vi "Main.vi"() -> ()   [LabVIEW 2013] (continued)
              tunnel: DB_-_[TransactionNo],[OrderNo]."h.[AdditionalProcs]" ("h.[TransactionNo],i.[OrderNo]\n2014-09-27 11:16") -> [w2623]
              tunnel: w2507 -> [w2613]
              tunnel: w2550 -> [w2622]
              tunnel: w2508 -> [w2606]
              tunnel: w2505 -> [w2604]
              tunnel: w2504 -> [w2602]
              tunnel: w2526 -> [w2621]
              tunnel: w2532 -> [w2620]
              tunnel: w2525 -> [w2619]
              tunnel: DB_-_[TransactionNo],[OrderNo]."h.[OutputSetId]" ("h.[TransactionNo],i.[OrderNo]\n2014-09-27 11:16") -> [w2616]
              tunnel: "Output Set" ("String") -> [w2611]
              tunnel: [w2610] -> w2518
              tunnel: w2501 -> [w2600]
              tunnel: [w2598] -> w2500 mode=indexing
              tunnel: w2499 -> [w2597]
              # "8"
              # "SpreadsheetString has \\r\\n\notherwise must add \\r\\n"
              # "6"
              # "4"
              # "7"
              # "Parameters"
              # "9"
              # "3"
              # "2"
              # "1"
              # "Each Order No"
              n1506 = for {
                tunnel: w2617 -> [w2657]
                tunnel: w2624 -> [w2656] mode=indexing
                shift-right: [w2651] -> w2615
                shift-left: w2597 -> [w2655]
                tunnel: w2621 -> [w2654] mode=indexing
                # "Part Details Columns"
                n1507 = Index Array(array=w2657, index=w2656) -> (element=w2653:string)
                n1508 = Build Array "Col0\nCol1"(w2654, w2653) -> (w2652:string[])
                n1509 = Build Array (concatenate) "New Row"(w2655, w2652) -> (w2651:string[][])
              }
              n1510 = Build Array (concatenate) "New Rows"(w2615, w2614, w2613) -> (w2612:string[][])
              n1511 = for {
                tunnel: w2617 -> [w2650]
                tunnel: w2622 -> [w2649] mode=indexing
                shift-right: [w2644] -> w2618
                shift-left: w2612 -> [w2646]
                tunnel: w2620 -> [w2648] mode=indexing
                # "WPS Column"
                n1512 = Index Array(array=w2650, index=w2649) -> (element=w2647:string)
                n1513 = Build Array "Col0\nCol1"(w2648, w2647) -> (w2645:string[])
                n1514 = Build Array (concatenate) "New Row"(w2646, w2645) -> (w2644:string[][])
              }
              n1515 = flat-sequence {
                tunnel: w2623 -> [w2636]
                tunnel: w2617 -> [w2635]
                tunnel: w2619 -> [w2634]
                tunnel: [w2631] -> w2609
                tunnel: w2618 -> [w2633]
                frame #0 {
                  # "5"
                  # "Additional WPS Column"
                  n1516 = Index Array(array=w2635, index=w2636) -> (element=w2630:string)
                  n1517 = Spreadsheet String To Array(delimiter (Tab)="\r\n", format string="", spreadsheet string=w2630, array type (2D Dbl)=string[] []) -> (array=w2626:string[])
                  n1518 = for {
                    tunnel: w2626 -> [w2639] mode=indexing
                    tunnel: [w2639] -> w2625 mode=indexing if=w2637
                    n1519 = Search and Replace String(replace all?=TRUE ("replace all? (F)"), input string=w2639, search string=",") -> (result string=w2641:string)  [unwired: 5 in, 3 out]
                    n1520 = call <vilib>:"Trim Whitespace.vi"("string"=w2641) -> ("trimmed string"=w2640:string)  [unwired: 1 in]
                    n1521 = Empty String/Path?(string/path=w2640) -> (empty?=w2638:bool)
                    n1522 = Not(x=w2638) -> (.not. x?=w2637:bool)
                  }
                  n1523 = Build Array (concatenate) "Col0\nCol1"(w2634, w2625) -> (w2632:string[])
                  n1524 = Build Array (concatenate) "New Row"(w2633, w2632) -> (w2631:string[][])
                }
              }
              n1525 = Index Array(array=w2617, index=w2616) -> (element=w2610:string)
              n1526 = Build Array "Col0\nCol1"(w2611, w2610) -> (w2608:string[])
              n1527 = Build Array (concatenate) "New Row"(w2609, w2608) -> (w2607:string[][])
              n1528 = Build Array (concatenate) "New Rows"(w2607, w2606) -> (w2605:string[][])
              n1529 = Build Array (concatenate) "New Row"(w2605, w2604) -> (w2603:string[][])
              n1530 = Build Array (concatenate) "New Row"(w2603, w2602) -> (w2601:string[][])
              n1531 = Build Array (concatenate) "New Row"(w2601, w2600) -> (w2599:string[][])
              n1532 = Flatten To String(anything=w2599) -> (data string=w2598:string)  [unwired: 3 in, 2 out]
            }
            n1533 = call "DB - [MasterData].[OutputSet].vi"("Master Data OuputSet SQL"=DB_-_Master_Data_OutputSet_SQL."SELECT [LayoutFilePath],[LayoutFileName]", "[PlantId]"=w2521, "[OutputSetId]"=w2518) -> ("Template Files"=w2517:string[], "[LayoutId]"=w2515:string[])  [unwired: 4 in, 3 out]
            n1534 = String To Path(string=w2517) -> (path=w2516:path[])
            n1535 = local write "DB"(w2533) -> ()
          }
        }
        "Order No" <- w2205
        "Details From .stp and Parameters" <- w2210
        n1536 = Array Size(array=w2205) -> (size(s)=w2206:i32)
        "No Of Orders" <- w2206
        n1537 = local read "DB - Report"() -> (w2199:bool)
        n1538 = Format Date/Time String "Date_Time"(time format string (%c)="%Y%m%d_%H%M%S") -> (date/time string=w2203:string)  [unwired: 2 in]
        n1539 = Format Into String(format string="%02d", w2206) -> (resulting string=w2201:string)  [unwired: 2 in, 1 out]
        n1540 = local read "Chart Separation by Order#"() -> (w2204:bool)
        n1541 = case shown="True" w2199 {
          tunnel: w2197 -> [_ w2379]
          tunnel: w2173 -> [_ w2377]
          tunnel: ["00" ("[ReportRunNo]") w2372] -> w2198
          tunnel: [w2356 w2361] -> w2172
          tunnel: [w2355 w2360] -> w2171
          frame False {
            # "Use Logon's INFO if no Database"
            n1542 = local read "Logon (Report Buffer)"() -> (w2357:T21)
            n1543 = Unbundle By Name(w2357) -> ("PlantID"=w2356:string, "SystemID"=w2355:string)
          }
          frame True {
            w2362 = 1  # [SystemId]
            w2363 = 0  # [PlantId]
            w2378 = ""  # Not Needed for [TransactionRunNo]
            # "[Execute].[TransactionReport] logged inside subVI"
            n1544 = Bundle("TransactionNo"=w2379, "Not Needed for [TransactionRunNo]"=w2378) -> (w2365:T67)  [unwired: 1 in]
            n1545 = call "DB - [Execute].[ReportList].vi"(2:DB_-_Execute_ReportList_Enum."INSERT INTO [Execute].[TransactionReport]", "Transaction"=w2365, "error in (no error)"=w2377) -> ("[ReportRunNo]"=w2373:string, "SUMMARY"=w2369:errorcluster)  [unwired: 9 in, 2 out]
            n1546 = Concatenate Strings("{Report Generate Toggle} [ReportRunNo] = " ("Message"), w2373) -> (w2370:string)
            n1547 = local read "Transaction (Report Buffer)"() -> (w2359:T19)
            n1548 = Decimal String To Number(string=w2373) -> (number=w2374:i32)  [unwired: 2 in, 1 out]
            n1549 = call "Queue - EnQueue to MessageQ.vi"("<NoD> Don't Display to UI"=TRUE, "Message"=w2370) -> ()  [unwired: 9 in, 1 out]
            n1550 = Format Into String(format string="%02d", w2374) -> (resulting string=w2372:string)  [unwired: 2 in, 1 out]
            n1551 = call "DB - [Setup].[Item] (Part Details).vi"("DB - Setup Item Enum"=DB_-_Setup_Item_Enum."SELECT [EquipmentxId]", "DB.Schema.Table Array"=string[] ["SRTRS.Execute.Header"], "Transaction"=w2359, "error in (no error)"=w2369) -> ("1D Results"=w2364:string[], "SUMMARY"=w2368:errorcluster)  [unwired: 6 in, 4 out]
            n1552 = Index Array(array=w2364, index #1=w2363, index #2=w2362) -> (element #1=w2361:string, element #2=w2360:string)
            n1553 = local write "DB"(w2368) -> ()
          }
        }
        n1554 = Concatenate Strings(w2201, w2198) -> (w2208:string)
        n1555 = Select(t=w2208, s=w2204, f=w2203) -> (s? t:f=w2202:string)
        n1556 = flat-sequence {
          tunnel: w2200 -> [w2352]
          tunnel: [w2352] -> w2196
          frame #0 {
            n1557 = call "Msgbox - Add OR Remove.vi"("MsgBox"=T44 {"Show"=FALSE, "Priority"=0, "Message"="Report Generation...(Done)", "seconds"=30}) -> ("Error Out"=→"Msgbox":errorcluster)  [unwired: 9 in, 1 out]
          }
        }
        n1558 = for {
          tunnel: [w2245] -> w2179 mode=concatenating
          tunnel: w2210 -> [w2244]
          tunnel: w2205 -> [w2243]
          tunnel: w2202 -> [w2242]
          tunnel: w2201 -> [w2241]
          tunnel: [w2240] -> w2193
          tunnel: w2198 -> [w2238]
          tunnel: w2197 -> [w2237]
          shift-right: [w2239] -> w2200
          shift-left: w2173 -> [w2235]
          tunnel: w2195 -> [w2234] mode=indexing
          tunnel: w2194 -> [w2233] mode=indexing
          tunnel: w2172 -> [w2232]
          tunnel: w2171 -> [w2231]
          i -> [w2236]
          # "Template Files"
          n1559 = local write "Template File"(w2234) -> ()
          n1560 = local write "Layout ID"(w2233) -> ()
          n1561 = for {
            tunnel: w2244 -> [w2284] mode=indexing
            tunnel: w2243 -> [w2268] mode=indexing
            tunnel: w2237 -> [w2269]
            tunnel: w2242 -> [w2286]
            shift-right: [w2283] -> w2239
            shift-left: w2235 -> [w2253]
            tunnel: [w2280] -> w2245 mode=indexing
            tunnel: w2238 -> [w2248]
            tunnel: w2241 -> [w2267]
            tunnel: [w2264] -> w2240
            tunnel: w2234 -> [w2262]
            tunnel: w2236 -> [w2258]
            tunnel: w2233 -> [w2260]
            tunnel: w2232 -> [w2247]
            tunnel: w2231 -> [w2246]
            i -> [w2259]
            w2282 = "\"" ("string")
            w2261 = "_" ("string")
            # "List by Order Number (Easier to maintain code if on seperate loop)"
            n1562 = Equal To 0?(x=w2258) -> (x = 0?=w2256:bool)
            n1563 = Equal To 0?(x=w2259) -> (x = 0?=w2257:bool)
            n1564 = And(x=w2257, y=w2256) -> (x .and. y?=w2255:bool)
            n1565 = local read "Excel"() -> (w2263:path)
            n1566 = local read "Reports"() -> (w2274:path)
            n1567 = Concatenate Strings(w2260, w2261, w2269, w2261, w2268, w2261, w2286, ".xls" ("string")) -> (w2254:string)
            n1568 = case shown="True" w2255 {
              frame True {
                n1569 = call "Msgbox - Add OR Remove.vi"("MsgBox"=T44 {"Show"=TRUE, "Priority"=0, "Message"="Report Generation...", "seconds"=30}) -> ("Error Out"=w2288:errorcluster)  [unwired: 9 in, 1 out]
                n1570 = local write "Msgbox"(w2288) -> ()
              }
              frame False {
              }
            }
            n1571 = call "Folder - Create Year-Month.vi"("error in (no error)"=w2253, "Folder Name"=w2274) -> ("error out"=w2276:errorcluster, "Folder with Year\\Month"=w2266:path)  [unwired: 8 in]
            n1572 = call "Folder - Create Year-Month.vi"("error in (no error)"=w2253, "Folder Name"=w2263) -> ("error out"=w2277:errorcluster, "Folder with Year\\Month"=w2278:path)  [unwired: 8 in]
            n1573 = Merge Errors(w2277, w2276) -> (w2279:errorcluster)
            n1574 = local read "MasterData\\JPG"() -> (w2273:path)
            n1575 = local read "Raw Data File (Report Tab)"() -> (w2265:path)
            n1576 = Build Path(base path=w2278, name or relative path=w2254) -> (appended path=w2272:path)
            n1577 = local read "Logon"() -> (w2252:T21)
            n1578 = Unbundle By Name(w2252) -> ("LanguageID"=w2250:string)
            n1579 = local read "Temp_Host"() -> (w2271:path)
            n1580 = Bundle By Name(cluster=T50 {"[LanguageId]"="", "[ReportRunNo]"="", "[PlantId]"="", "[SystemId]"=""} ("Report Additional Details"), "[LanguageId]"=w2250, "[ReportRunNo]"=w2248, "[PlantId]"=w2247, "[SystemId]"=w2246) -> (w2249:T50)
            n1581 = Bundle("Reports"=w2274, "MasterData\\JPG"=w2273, "String"=w2262, "appended path"=w2272, "Raw Data File (Report Tab)"=w2265, "Temp_Host"=w2271) -> (w2270:T68)  [unwired: 1 in]
            "Report Files Cluster" <- w2270
            n1582 = while {
              tunnel: w2284 -> [w2302]
              tunnel: [w2297] -> w2283
              tunnel: w2279 -> [w2301]
              tunnel: w2270 -> [w2296]
              tunnel: w2249 -> [w2291]
              i -> [w2298]
              stop <- w2299 stop-if-true
              # "Try twice or no error"
              n1583 = local read "Chart Separation by Order#"() -> (w2294:bool)
              n1584 = local read "DB - Report"() -> (w2295:bool)
              n1585 = call "Report - Excel.vi"("pdf"="Report.Create.PDF", "Chart Seperation by Order#"=w2294, "Details from .stp and Parameters"=w2302, "Use DB for Picture (Material)"=w2295, "error in (no error)"=w2301, "Include MetaData"="Include MetaData", "Report Additional Details"=w2291, "Report Files Cluster"=w2296) -> ("error out"=w2300:errorcluster, "Picture Error"=w2290:errorcluster, "Material File"=w2289:string)  [unwired: 1 in]
              n1586 = case shown="Error" w2290 {
                tunnel: w2289 -> [_ w2303]
                frame No Error {
                }
                frame Error {
                  n1587 = Concatenate Strings("{Report} Pic Error:  " ("Message"), w2303) -> (w2304:string)
                  n1588 = call "Queue - EnQueue to MessageQ.vi"("<NoD> Don't Display to UI"=TRUE, "Message"=w2304) -> ()  [unwired: 9 in, 1 out]
                }
              }
              n1589 = case shown="Error" w2300 {
                selector: w2300 -> [w2307 w2309]
                tunnel: [TRUE w2310] -> w2299
                tunnel: w2298 -> [_ w2312]
                tunnel: [w2307 w2311] -> w2297
                frame No Error {
                }
                frame Error {
                  n1590 = Greater Or Equal?(x=w2312, y=2) -> (x >= y?=w2310:bool)
                  n1591 = case shown="True" w2310 {
                    tunnel: [errorcluster {"status"=FALSE, "code"=0, "source"=""} ("error out") w2315] -> w2311
                    tunnel: w2309 -> [_ w2315]
                    frame False {
                    }
                    frame True {
                    }
                  }
                }
              }
            }
            n1592 = Concatenate Strings(w2282, w2254, w2282) -> (w2281:string)
            n1593 = case shown="No Error" w2283 {
              tunnel: [_ " create ERROR." ("string")] -> w2275
              tunnel: w2268 -> [w2337 _]
              tunnel: w2248 -> [w2336 _]
              tunnel: w2267 -> [w2335 _]
              tunnel: w2266 -> [w2334 _]
              tunnel: w2265 -> [w2333 _]
              tunnel: [w2332 errorcluster {"status"=FALSE, "code"=0, "source"=""} ("SUMMARY")] -> w2264
              tunnel: w2254 -> [w2318 _]
              tunnel: w2260 -> [w2316 _]
              frame No Error {
                # "Use Logon or From Execute.Setup.Header?"
                n1594 = Search and Replace String(replace all?=TRUE ("replace all? (F)"), case sensitive?=TRUE ("ignore case? (F)"), input string=w2318, search string="xls", replace string="pdf" ("replace string (\"\")")) -> (result string=w2317:string)  [unwired: 3 in, 3 out]
                n1595 = Strip Path(path=w2333) -> (stripped path=w2324:path, name=w2323:string)
                n1596 = Path To String(path=w2334) -> (string=w2329:string)
                n1597 = Path To String(path=w2324) -> (string=w2325:string)
                n1598 = local read "ReportList Cluster"() -> (w2327:T18)
                n1599 = Bundle By Name(cluster=w2327, "[LayoutId]"=w2316, "[OrderNo]"=w2337, "[ReportRunNo]"=w2336, "[NoOfOrders]"=w2335, "[ReportFilePath]"=w2329, "[ReportFileName]"=w2317, "[RawDataSourcePath]"=w2325, "[RawDataSourceFileName]"=w2323) -> (w2328:T18)
                "ReportList Cluster" <- w2328
                n1600 = local read "Transaction (Report Buffer)"() -> (w2330:T19)
                n1601 = local read "Logon (Report Buffer)"() -> (w2326:T21)
                n1602 = call "DB - [Execute].[ReportList].vi"(2:DB_-_Execute_ReportList_Enum."INSERT INTO [Execute].[ReportList] ", "Transaction"=w2330, "ReportList Cluster"=w2328, "Logon"=w2326) -> ("SUMMARY"=w2332:errorcluster)  [unwired: 8 in, 3 out]
                n1603 = local write "DB"(w2332) -> ()
              }
              frame Error {
              }
            }
            n1604 = Concatenate Strings(w2281, w2275) -> (w2280:string)
          }
        }
        n1605 = case shown="True" w2199 {
          tunnel: w2200 -> [_ w2340]
          tunnel: w2198 -> [_ w2342]
          tunnel: w2197 -> [_ w2341]
          frame False {
            # "Skip DB"
          }
          frame True {
            # "Use DB - Update [ReportGenerateFail] Flag if Report Fail"
            n1606 = case shown="Error" w2340 {
              tunnel: w2342 -> [_ w2348]
              tunnel: w2341 -> [_ w2347]
              frame No Error {
              }
              frame Error {
                n1607 = Bundle("TransactionNo"=w2347, "") -> (w2345:cluster{"TransactionNo":string, string})  [unwired: 1 in]
                n1608 = call "DB - [Execute].[ReportList].vi"(2:DB_-_Execute_ReportList_Enum."UPDATE [Execute].[TransactionReport]", "[ReportGenerateFail]"=TRUE, "[ReportRunNo]"=w2348, "Transaction"=w2345) -> ("SUMMARY"=w2349:errorcluster)  [unwired: 8 in, 3 out]
                n1609 = local write "DB"(w2349) -> ()
              }
            }
          }
        }
        n1610 = Array To Spreadsheet String(delimiter (Tab)=", ", array=w2179, 3:"" ("format string")) -> (spreadsheet string=w2183:string)
        n1611 = Search and Replace String(replace all?=TRUE ("replace all? (F)"), case sensitive?=TRUE ("ignore case? (F)"), input string=w2183, search string="xls", replace string="pdf" ("replace string (\"\")")) -> (result string=w2182:string)  [unwired: 3 in, 3 out]
        n1612 = Search and Replace String(replace all?=TRUE ("replace all? (F)"), input string=w2182, search string="\r\n") -> (result string=w2178:string)  [unwired: 5 in, 3 out]
        n1613 = case shown="Error" w2196 {
          selector: w2196 -> [_ w2666]
          tunnel: ["<I 405>" ("<.?....> Message Code") "<E 406>" ("<.?....> Message Code")] -> w2192
          tunnel: ["Report Generate Successful" ("<.?....> Message Code") "Report Generate Fail" ("<.?....> Message Code")] -> w2191
          tunnel: [" report(s) Generated" ("<.?....> Message Code") "Please check output set and file server availability and Retry." ("<.?....> Message Code")] -> w2190
          tunnel: w2178 -> [w2658 _]
          tunnel: [w2658 _] -> w2177
          frame No Error {
            # "Report Generated OK!"
          }
          frame Error {
            # "Report Generate Failed."
            n1614 = Unbundle By Name(w2666) -> ("code"=w2665:i32)
            n1615 = case shown="0, Default" w2665 {
              tunnel: w2666 -> [_ _]
              frame 0, Default {
              }
              frame -8001 {
                # "Repeat?"
                # "Error Popup already shown\nearlier"
              }
            }
          }
        }
        n1616 = call "Msgbox - Message Handler.vi"("Short Description (When DB Not Available)"=w2191, "Description (When DB Not Available)"=w2190, "Pre-Description"=w2177, "<.?....> Message Code"=w2192) -> ("MHandler Error"=w2174:errorcluster)  [unwired: 5 in, 2 out]
        n1617 = local write "MHandler"(w2174) -> ()
        n1618 = case shown="No Error" w2193 {
          tunnel: ["<NoD>INSERT INTO [Execute].[ReportList]" ("Message") "Report List DB Error. /*INSERT [EXECUTE].[ReportList]*/" ("Message")] -> w2176
          frame No Error {
            # "No Need to Display this in Message."
          }
          frame Error {
          }
        }
        n1619 = call "Queue - EnQueue to MessageQ.vi"("<NoD> Don't Display to UI"=TRUE, "Message"=w2176) -> ()  [unwired: 9 in, 1 out]
        n1620 = flat-sequence {
          tunnel: w2193 -> [_]
          frame #0 {
            n1621 = local read "Template File"() -> (w2219:path)
            n1622 = local read "Layout ID"() -> (w2217:string)
            n1623 = Path To String(path=w2219) -> (string=w2216:string)
            n1624 = call <vilib>:"Application Directory.vi"() -> ("Application Directory"=w2224:path)
            n1625 = Concatenate Strings(w2217, "\t", w2216) -> (w2215:string)
            n1626 = Build Path(base path=w2224, name or relative path="SRTRS.ini" ("ini Name")) -> (appended path=w2223:path)
            n1627 = call <vilib>:"Open Config Data.vi"("create file if necessary (T)"=FALSE, "configuration file path"=w2223) -> ("error out"=w2226:errorcluster, "refnum"=w2225:T59)  [unwired: 7 in, 1 out]
            n1628 = call-poly <vilib>:"Write Key.vi"("write raw string? (F)"=TRUE, "section"="Settings", "error in (no error)"=w2226, "value"=w2215, "key"="Layout Details", "refnum"=w2225) -> ("error out"=w2230:errorcluster, "refnum out"=w2229:T59)  [unwired: 3 in, 1 out]
            n1629 = call <vilib>:"Close Config Data.vi"("error in (no error)"=w2230, "refnum"=w2229) -> ("error out"=w2228:errorcluster)  [unwired: 8 in, 1 out]
            n1630 = local write "ini File Error"(w2228) -> ()
          }
        }
      }
      event "------------------------------------        Simulate TAB      ------------------------------------": Value Change {
        n1631 = event-data() -> ()  [unwired: 1 in, 6 out]
      }
      event "Use Host COM Port": Value Change {
        # "Set COM Port to either Local PC or via cRIO"
        n1632 = event-data() -> ("CtlRef"=w2678:refnum<vi>)  [unwired: 1 in, 5 out]
        n1633 = property class="Bool (strict)"(reference=w2678) -> ("Label.Text"=w2676:string)  [unwired: 1 in, 2 out]
        n1634 = local read "Host COM Port"() -> (w2681:string)
        n1635 = local read "cRIO COM Port"() -> (w2680:string)
        n1636 = Select(t="TRUE.", s="Use Host COM Port", f="FALSE.") -> (s? t:f=w2671:string)
        n1637 = Concatenate Strings("{[" ("string"), w2676, "]}" ("string")) -> (w2674:string)
        n1638 = Select(t=w2681, s="Use Host COM Port", f=w2680) -> (s? t:f=w2679:string)
        n1639 = Concatenate Strings(w2674, " is Changed to " ("string"), w2671) -> (w2668:string)
        n1640 = local write "VISA resource name RS232"(w2679) -> ()
        n1641 = call "Queue - EnQueue to MessageQ.vi"("<NoD> Don't Display to UI"=TRUE, "Message"=w2668) -> ()  [unwired: 9 in, 1 out]
      }
      event "Simulate cRIO Started": Value Change {
        # "Seq Num        Ramp Rate       Target Temp        SegType"
        n1642 = event-data() -> ()  [unwired: 1 in, 6 out]
        n1643 = case shown="False" FALSE {
          tunnel: [100 ("Start Temp") 25 ("Start Temp")] -> w2685
          tunnel: [i32[][] [[2, 0, 0, 3], [3, 50, 80, 1], [4, 0, 0, 0]] ("Final Segments") i32[][] [[1, 100, 100, 1], [2, 0, 0, 3], [3, 50, 80, 1], [4, 0, 0, 0]] ("Final Segments")] -> w2684
          frame False {
            # "From Hold at 100° to Ramp Down"
          }
          frame True {
            # "All Segments (Ramp Up, Hold, Ramp Down)"
          }
        }
        n1644 = local read "cRIO shared variable RT Library"() -> (w2682:string)
        n1645 = control-ref of="cRIO Status"() -> (w2688:refnum<vi>)
        n1646 = call "cRIO - Shared Variable RW.vi"("shared variable RT Library"=w2682, "Read/Write"=cRIO_RW_Enum."Write", "Simulate cRIO"=TRUE, "Probe List In"=i32[] [1, 2], "DAQ Start"=TRUE, "cRIO Status"=w2688) -> ()  [unwired: 5 in, 9 out]
        n1647 = call "ET3500 - Simulate Profile.vi"("Popup"=FALSE, "Set (T) / Get (F)"=TRUE, "Start Temp"=w2685, "Final Segments"=w2684) -> ()  [unwired: 3 in, 5 out]
      }
      event "Data", "Excel", "Report.Create.Excel", "Report.Create.PDF", "Simulate cRIO", "Simulate ET3500": Value Change {
        # "<OPTIONS> are logged into MessageQ"
        n1648 = event-data() -> ("CtlRef"=w2706:refnum<vi>)  [unwired: 1 in, 5 out]
        n1649 = property class="Ctl"(reference=w2706) -> ("ClassName"=w2699:string, "Caption.Text"=w2700:string, "Value"=w2704:variant)  [unwired: 1 in, 2 out]
        n1650 = case shown="\"Boolean\"" w2699 {
          tunnel: w2704 -> [w2712 w2718]
          tunnel: [w2707 w2713] -> w2703
          frame "Path", Default {
            w2708 = "\"" ("string")
            n1651 = Variant To Data(type=path "", Variant=w2712) -> (data=w2710:path)  [unwired: 1 in, 1 out]
            n1652 = Path To String(path=w2710) -> (string=w2709:string)
            n1653 = Concatenate Strings(w2708, w2709, w2708) -> (w2707:string)
          }
          frame "Boolean" {
            n1654 = Variant To Data(type=TRUE, Variant=w2718) -> (data=w2716:bool)  [unwired: 1 in, 1 out]
            n1655 = Select(t="TRUE" ("string"), s=w2716, f="FALSE" ("string")) -> (s? t:f=w2713:string)
          }
        }
        n1656 = Concatenate Strings("<", w2700, ">", " changed to " ("string"), w2703) -> (w2698:string)
        n1657 = call "Queue - EnQueue to MessageQ.vi"("<NoD> Don't Display to UI"=TRUE, "Message"=w2698) -> ()  [unwired: 9 in, 1 out]
      }
      event "------------------------------------        MCListBox       ------------------------------------": Value Change {
        n1658 = event-data() -> ()  [unwired: 1 in, 6 out]
      }
      event "MCListBox FHS Setup Add Button", "MCListBox FHS Setup Remove Button", "MCListBox AWPS Add Button", "MCListBox AWPS Remove Button", "MCListBox FHS Master Data Add Button", "MCListBox FHS Master Data Remove Button": Value Change {
        # "New and Unsed Cells have same color for\nAWPS but different color for FHS Master Data"
        # "Not in used"
        n1659 = event-data() -> ("CtlRef"=w2733:refnum<vi>)  [unwired: 1 in, 5 out]
        n1660 = local read "CellBG Unused Cells"() -> (w2725:u32)
        n1661 = local read "CellBG New Cells"() -> (w2726:u32)
        n1662 = Or(x="MCListBox FHS Master Data Add Button", y="MCListBox FHS Master Data Remove Button") -> (x .or. y?=w2720:bool)
        n1663 = Or(x="MCListBox FHS Setup Add Button", y="MCListBox FHS Setup Remove Button") -> (x .or. y?=w2721:bool)
        n1664 = Or(x=w2721, y=w2720) -> (x .or. y?=w2719:bool)
        n1665 = Select(t=w2726, s=w2719, f=w2725) -> (s? t:f=w2724:u32)
        n1666 = case shown="True" "MCListBox AWPS Add Button" {
          tunnel: [T5[] [] w2753] -> w2732
          tunnel: [_ w2752] -> w2730
          frame False {
          }
          frame True {
            w2747 = ""
            # "To Add via ComboBox"
            n1667 = control-ref of="Additional Rev"() -> (w2754:refnum<vi>)
            n1668 = control-ref of="Additional WPS/Ref"() -> (w2755:refnum<vi>)
            n1669 = control-ref of="MCListBox AWPS"() -> (w2746:refnum<vi>)
            n1670 = property class="MCListbox (strict)"(reference=w2746) -> ("ItemNames"=w2745:string[][])  [unwired: 1 in, 2 out]
            n1671 = property class="CmbBox (strict)"(reference=w2755) -> (reference out=w2749:refnum<vi>, "Value"=w2743:T5)  [unwired: 1 in, 1 out]
            n1672 = property class="CmbBox (strict)"(reference=w2754) -> (reference out=w2748:refnum<vi>, "Value"=w2736:T5)  [unwired: 1 in, 1 out]
            n1673 = Array To Spreadsheet String(array=w2745, 3:"" ("format string")) -> (spreadsheet string=w2739:string)  [unwired: 1 in]
            n1674 = Empty String/Path?(string/path=w2736) -> (empty?=w2750:bool)
            n1675 = call <vilib>:"Space Constant.vi"() -> ("String"=w2735:string)
            n1676 = Select(t=w2735, s=w2750, f=w2736) -> (s? t:f=w2741:T5)
            n1677 = Empty String/Path?(string/path=w2743) -> (empty?=w2751:bool)
            n1678 = Concatenate Strings(w2743, "\\t", w2741) -> (w2740:string)
            n1679 = Match Pattern(string=w2739, regular expression=w2740) -> (offset past match=w2738:i32)  [unwired: 1 in, 3 out]
            n1680 = Greater Or Equal To 0?(x=w2738) -> (x >= 0?=w2737:bool)
            n1681 = Build Array(w2743, w2741) -> (w2753:T5[])
            n1682 = case shown="True" w2751 {
              tunnel: [w2756 errorcluster {"status"=TRUE, "code"=0, "source"=""} ("error constant")] -> w2752
              tunnel: w2737 -> [w2757 _]
              frame False {
                # "Not Empty Field"
                n1683 = case shown="True" w2757 {
                  tunnel: [_ errorcluster {"status"=TRUE, "code"=0, "source"=""} ("error constant")] -> w2756
                  frame False {
                  }
                  frame True {
                    # "Addtional WPS and Rev already Exists in AWPS MCListBox"
                    n1684 = call "Msgbox - Format Message.vi"("Message"="Duplicates. Additional WPS/Ref and Rev are not Added." ("message"), "Message Code\n2014-10-01"=Message_Code_-_Enum."<APP><W 130>" ("Message Code\n2014-10-01")) -> ("Message"=w2760:string)  [unwired: 8 in, 1 out]
                    n1685 = call "Msgbox UI.vi"("[MessageType]"=w2760) -> ()  [unwired: 8 in, 3 out]
                  }
                }
              }
              frame True {
                # "Empty Field"
                n1686 = call "Msgbox - Format Message.vi"("Message"="Empty Field. Additional WPS/Ref and Rev are not Added." ("message"), "Message Code\n2014-10-01"=Message_Code_-_Enum."<APP><W 130>" ("Message Code\n2014-10-01")) -> ("Message"=w2764:string)  [unwired: 8 in, 1 out]
                n1687 = call "Msgbox UI.vi"("[MessageType]"=w2764) -> ()  [unwired: 8 in, 3 out]
              }
            }
            n1688 = property class="CmbBox (strict)"(reference=w2749, "Value"=w2747) -> ()  [unwired: 1 in, 2 out]
            n1689 = property class="CmbBox (strict)"(reference=w2748, "Value"=w2747) -> ()  [unwired: 1 in, 2 out]
          }
        }
        n1690 = call "MCListbox Event - Add and Remove Buttons.vi"("CellBG New Cells"=w2724, "CellBG Unused Cells"=w2725, "new element/subarray"=w2732, "Error In"=w2730, "MCListBox Ref"=w2731, "CtlRef Boolean"=w2733) -> ()  [unwired: 5 in, 1 out]
      }
      event "MCListBox FHS Setup", "MCListBox FHS Master Data": Key Down? {
        # "Only the 2 FHS (Furnace Heating Sequence) have direct Keyboard Entries"
        n1691 = event-data() -> ("CtlRef"=w2767:refnum<vi>, "Char"=w2768:i16, "VKey"=w2770:T55)  [unwired: 1 in, 7 out]
        n1692 = property class="MCListbox (strict)"(reference=w2767) -> ("EditPos"=w2766:T33)  [unwired: 1 in, 2 out]
        n1693 = call "MCListbox Event - Key Down QuestionMark.vi"("Key Down?"=w2772, "CtlRef"=w2767) -> ()  [unwired: 9 in, 1 out]
        n1694 = case "Only NUMBERS, BackSpace and (Return, Enter, Up, Down, Right, Left, Delete)" shown="8, 46, 48..57" w2768 {
          tunnel: [w2774 w2777 w2778] -> w2769
          tunnel: w2770 -> [w2773 _ _]
          tunnel: w2766 -> [_ _ w2779]
          frame 0, Default {
            # "Exception"
            n1695 = case shown="\"Enter\", \"Return\", \"Up\"..\"Right\", \"Delete\"" w2773 {
              tunnel: [w2775 w2776] -> w2774
              frame Default {
                w2775 = TRUE  # Discard
              }
              frame "Enter", "Return", "Up".."Right", "Delete" {
                w2776 = FALSE  # Do Not Discard
                # "Up, Down, Left, Right, Delete"
              }
            }
          }
          frame 8, 46, 48..57 {
            w2777 = FALSE  # Do not discard
            # "Char\n46        .     (decimal Point)\n48-57  0-9 (Numbers)\n58        :      (colon)\n8          Backspace"
            # "Backspace, decimal point, Numbers, colon"
          }
          frame 58 {
            w2780 = 3  # Hold Time Column
            # "Discard if not Hold Time Column"
            # "Char\n46        .     (decimal Point)\n48-57  0-9 (Numbers)\n58        :      (colon)\n8          Backspace"
            n1696 = Unbundle By Name(w2779) -> ("Column"=w2781:i32)
            n1697 = Not Equal?(x=w2781, y=w2780) -> (x != y?=w2778:bool)
          }
        }
        n1698 = event-data("Discard?"=w2769) -> ()  [unwired: 1 in, 1 out]
      }
      event "MCListBox FHS Setup", "MCListBox FHS Master Data": Key Down {
        w2786 = i16 9  # TAB
        # "Only the 2 FHS (Furnace Heating Sequence) have direct Keyboard Entries"
        n1699 = event-data() -> ("CtlRef"=w2794:refnum<vi>, "Char"=w2787:i16, "VKey"=w2789:T55)  [unwired: 1 in, 7 out]
        n1700 = call "MCListbox Event - Key Down.vi"("VKey"=w2789, "Char"=w2787, "CtlRef"=w2794) -> ("Edit Position B4 <RETURN>"=w2793:cluster{"row":i32, "col":i32})  [unwired: 7 in, 1 out]
        n1701 = Unbundle By Name(w2793) -> ("row"=w2792:i32, "col"=w2791:i32)
        n1702 = Equal?(x=eventvkey."Return", y=w2789) -> (x = y?=w2783:bool)
        n1703 = Equal?(x=eventvkey."Enter", y=w2789) -> (x = y?=w2784:bool)
        n1704 = Equal?(x=w2786, y=w2787) -> (x = y?=w2785:bool)
        n1705 = Compound Arithmetic op=OR(w2785, w2784, w2783) -> (w2782:bool)
        n1706 = case shown="True" w2782 {
          tunnel: w2794 -> [_ w2797]
          tunnel: w2791 -> [_ w2796]
          tunnel: w2792 -> [_ w2795]
          frame False {
          }
          frame True {
            # "Enter, Return"
            n1707 = case shown="1, 2" w2796 {
              selector: w2796 -> [_ w2805 w2814]
              tunnel: w2795 -> [_ w2806 w2815]
              tunnel: w2797 -> [_ w2799 w2811]
              frame 0, Default {
              }
              frame 3 {
                # "Hold Time Column"
                n1708 = property class="MCListbox (strict)"(reference=w2799) -> (reference out=w2800:refnum<vi>, "ItemNames"=w2798:string[][])  [unwired: 1 in, 1 out]
                n1709 = Index Array(array=w2798, index (row)=w2806, index (col)=w2805) -> (element=w2803:string)
                n1710 = call "String - Format to (HH_colon_MM).vi"("upper limit (Default 23 Hours)"=23, "xx:xx"=w2803) -> ("(HH:mm)"=w2802:string)  [unwired: 8 in, 1 out]
                n1711 = Replace Array Subset(array=w2798, new element=w2802, index (row)=w2806, index (col)=w2805) -> (w2804:string[][])
                n1712 = property class="MCListbox (strict)"(reference=w2800, "ItemNames"=w2804) -> ()  [unwired: 1 in, 2 out]
              }
              frame 1, 2 {
                # "Only allow for Decimal (floating point will be converted)"
                # "Ramp Rate, Target Temperature Column"
                n1713 = property class="MCListbox (strict)"(reference=w2811) -> (reference out=w2812:refnum<vi>, "ItemNames"=w2810:string[][])  [unwired: 1 in, 1 out]
                n1714 = Index Array(array=w2810, index (row)=w2815, index (col)=w2814) -> (element=w2809:string)
                n1715 = Fract/Exp String To Number(string=w2809) -> (number=w2807:dbl)  [unwired: 3 in, 1 out]
                n1716 = Number To Decimal String(number=w2807) -> (decimal integer string=w2808:string)  [unwired: 1 in]
                n1717 = Replace Array Subset(array=w2810, new element=w2808, index (row)=w2815, index (col)=w2814) -> (w2813:string[][])
                n1718 = property class="MCListbox (strict)"(reference=w2812, "ItemNames"=w2813) -> ()  [unwired: 1 in, 2 out]
              }
            }
          }
        }
      }
      event "MCListBox AWPS", "MCListBox FHS Setup", "MCListBox FHS Master Data": Mouse Down {
        # "Only the 2 FHS (Furnace Heating Sequence) AND AWPS  have selection of Row Cells Keyboard"
        n1719 = event-data() -> ("CtlRef"=w2816:refnum<vi>)  [unwired: 1 in, 7 out]
        n1720 = call "MCListbox Event - Mouse Down.vi"("CtlRef"=w2816) -> ()  [unwired: 10 in, 1 out]
      }
      event "------------------------------------        Part Details       ------------------------------------": Value Change {
        n1721 = event-data() -> ()  [unwired: 1 in, 6 out]
      }
      event "Part Details Add": Value Change {
        w2834 = string[] ["Order No.", "Oper. No.", "Qty.", "NCR No.", "Customer No.", "Customer Name", "Project", "Sales Order", "Item No.", "Material", "Revision", "Material Description", "Serial No.", "UnitOfQty"]  # 2014-10-17 08:39 Item Details Label.Text
        w2833 = string[] ["OrderNo", "OperationNo", "Qty", "NCRNo", "CustomerID", "Customer", "Project", "SalesOrderNo", "SalesOrderItemNo", "MaterialNo", "MaterialRev", "MaterialDesc", "SerialNos", "UnitOfQty"]  # 2014-10-17 08:39 [Config].[Mapping].[ColumnName]
        w2843 = string[] ["TC1", "TC2", "TC3", "TC4", "TC5", "TC6"]  # Channel to Probe Cluster Label
        # "Add new empty row to \nend of array"
        # "Checks for Mandatory Fields\nCalled by \"Item Details\", \"Channel Mapping\", \"Notes\", \"Plot\" Value Change"
        n1722 = event-data() -> ()  [unwired: 1 in, 6 out]
        n1723 = control-ref of="Plot"() -> (w2837:refnum<vi>)
        n1724 = control-ref of="Channel Mapping"() -> (w2861:refnum<vi>)
        n1725 = control-ref of="Item Details"() -> (w2864:refnum<vi>)
        n1726 = control-ref of="Channel to Probe Mapping"() -> (w2846:refnum<vi>)
        n1727 = property on="Part Details" class="MCListbox (strict)"() -> ("ColHdrString"=w2844:string[], "ItemNames"=w2850:string[][])  [unwired: 2 in, 2 out]
        n1728 = Array Size(array=w2844) -> (size(s)=w2858:i32)
        n1729 = Initialize Array("", w2858) -> (w2856:string[])
        n1730 = property class="Clust (strict)"(reference=w2861) -> ("Controls[]"=w2860:refnum<vi>[])  [unwired: 1 in, 2 out]
        n1731 = property class="Clust (strict)"(reference=w2864) -> ("Controls[]"=w2848:refnum<vi>[])  [unwired: 1 in, 2 out]
        n1732 = property class="Clust (strict)"(reference=w2837) -> ("Controls[]"=w2836:refnum<vi>[])  [unwired: 1 in, 2 out]
        n1733 = flat-sequence {
          frame #0 {
            n1734 = Wait (ms)(milliseconds to wait=u32 100) -> ()  [unwired: 1 out]
          }
          frame #1 {
            n1735 = local write "Part Details Add"(FALSE ("Part Details Add")) -> ()
          }
        }
        n1736 = control-ref of="No."() -> (w2849:refnum<vi>)
        n1737 = control-ref of="User"() -> (w2855:refnum<vi>)
        n1738 = control-ref of="Notes"() -> (w2847:refnum<vi>)
        n1739 = Index Array(array=w2850, index (col)=0 ("disabled index (col)")) -> (element=w2853:string[])  [unwired: 1 in]
        n1740 = Number To Decimal String(number="No.") -> (decimal integer string=w2851:string)  [unwired: 1 in]
        n1741 = Build Array (concatenate)(w2855, w2849, w2848, w2847, w2860, w2846, w2836) -> (w2862:refnum<vi>[])
        n1742 = Search 1D Array(1D array=w2853, element=w2851) -> (index of element=w2845:i32)  [unwired: 1 in]
        n1743 = case shown="-1" w2845 {
          selector: w2845 -> [w2965 _]
          tunnel: [w2965 w2970] -> w2863
          tunnel: [w2966 w2969] -> w2859
          tunnel: w2856 -> [_ w2968]
          tunnel: w2850 -> [w2966 w2967]
          frame 0, Default {
            # "Found"
          }
          frame -1 {
            # "last row"
            # "Not Found, Add new row"
            n1744 = Build Array (concatenate)(w2967, w2968) -> (w2969:string[][])
            n1745 = Array Size(array=w2969) -> (size(s)=w2972:i32[])
            n1746 = Index Array(array=w2972) -> (element=w2971:i32)  [unwired: 1 in]
            n1747 = Decrement(x=w2971) -> (x-1=w2970:i32)
          }
        }
        n1748 = local read "DB - Setup Item (Part Details)"() -> (w2835:bool)
        n1749 = case shown="False" w2835 {
          tunnel: [w2928 w2929] -> w2838
          frame False {
            w2928 = string[] ["Order No.", "Oper. No.", "Customer Name", "Project", "Material", "Material Description", "User"]  # Mandatory Fields Item Details Label.Text
          }
          frame True {
            n1750 = local read "[IsMandatory]\nLabel.Text"() -> (w2929:string[])
          }
        }
        n1751 = Array Size(array=w2838) -> (size(s)=w2831:i32)
        n1752 = for {
          tunnel: w2862 -> [w2984] mode=indexing
          tunnel: w2844 -> [w2982]
          shift-right: [w2977] -> w2823
          shift-left: w2859 -> [w2979]
          tunnel: w2863 -> [w2978]
          tunnel: w2834 -> [w2976]
          tunnel: w2833 -> [w2974]
          tunnel: w2828 -> [_]
          # "Match Ctl's Label Text to MClistBox Col Hdr[]"
          # "Find Match"
          # "Updates to MCListBox"
          n1753 = property class="Ctl"(reference=w2984) -> (reference out=w2973:refnum<vi>, "ClassName"=w2981:string, "Label.Text"=w2975:string, "Value"=w2983:variant)  [unwired: 1 in, 1 out]
          n1754 = Search 1D Array(1D array=w2982, element=w2975) -> (index of element=w2980:i32)  [unwired: 1 in]
          n1755 = case shown="0, Default" w2980 {
            selector: w2980 -> [w3002 _]
            tunnel: w2983 -> [w3004 _]
            tunnel: w2981 -> [w2990 _]
            tunnel: w2979 -> [w3003 w3068]
            tunnel: w2978 -> [w3001 _]
            tunnel: [w3000 w3068] -> w2977
            tunnel: w2976 -> [w2999 _]
            tunnel: w2975 -> [w2998 _]
            tunnel: w2974 -> [w2994 _]
            tunnel: [w2991 _] -> _
            tunnel: w2973 -> [w2989 _]
            frame 0, Default {
              # "Found Matching ColHdr[] In MCListBox"
              n1756 = case shown="\"Boolean\"" w2990 {
                tunnel: w3004 -> [w3060 w3063 w3067]
                tunnel: [w3057 w3061 w3064] -> w2992
                frame "Digital" {
                  n1757 = Variant To Data(type=0, Variant=w3060) -> (data=w3058:i32)  [unwired: 1 in, 1 out]
                  n1758 = Format Into String(w3058) -> (resulting string=w3057:string)  [unwired: 3 in, 1 out]
                }
                frame "ComboBox", "String", Default {
                  n1759 = Variant To Data(type="", Variant=w3063) -> (data=w3061:string)  [unwired: 1 in, 1 out]
                }
                frame "Boolean" {
                  n1760 = Variant To Data(type=TRUE, Variant=w3067) -> (data=w3065:bool)  [unwired: 1 in, 1 out]
                  n1761 = Format Into String(w3065) -> (resulting string=w3064:string)  [unwired: 3 in, 1 out]
                }
              }
              n1762 = local read "DB - Setup Item (Part Details)"() -> (w2996:bool)
              n1763 = Search 1D Array(1D array=w2999, element=w2998) -> (index of element=w2993:i32)  [unwired: 1 in]
              n1764 = Greater Or Equal To 0?(x=w2993) -> (x >= 0?=w2997:bool)
              n1765 = And(x=w2997, y=w2996) -> (x .and. y?=w2995:bool)
              n1766 = case shown="True" w2995 {
                tunnel: w2994 -> [w3029 _]
                tunnel: w2993 -> [w3028 _]
                tunnel: w2992 -> [w3026 w3056]
                tunnel: [w3025 w3056] -> w2988
                tunnel: [w3024 _] -> w2991
                tunnel: w2989 -> [w3023 _]
                tunnel: w2990 -> [w3022 _]
                frame True {
                  # "Found Label.Text's DB [ColumnName]. Resize Length Accordingly."
                  n1767 = Index Array "Get Matching ColumnName"(array=w3029, index=w3028) -> (element=w3021:string)
                  n1768 = local read "[Setup].[Item] COLUMN_NAME"() -> (w3027:string[])
                  n1769 = Search 1D Array(1D array=w3027, element=w3021) -> (index of element=w3024:i32)  [unwired: 1 in]
                  n1770 = case shown="0, Default" w3024 {
                    selector: w3024 -> [w3037 _]
                    tunnel: w3026 -> [w3035 w3055]
                    tunnel: [w3030 w3055] -> w3025
                    tunnel: w3023 -> [w3031 _]
                    tunnel: w3022 -> [w3032 _]
                    tunnel: w3021 -> [_ _]
                    frame 0, Default {
                      # "Get Column INFO from Local Variables set by \"DB - Column INFO.vi\" in Logon State"
                      n1771 = local read "[Setup].[Item] PRECISION"() -> (w3039:string[])
                      n1772 = Index Array(array=w3039, index=w3037) -> (element=w3034:string)
                      n1773 = Decimal String To Number(string=w3034) -> (number=w3033:i32)  [unwired: 2 in, 1 out]
                      n1774 = local read "[Setup].[Item] DATA_TYPE"() -> (w3038:string[])
                      n1775 = Index Array(array=w3038, index=w3037) -> (element=w3036:string)
                      n1776 = case shown="\"nvarchar\", Default" w3036 {
                        tunnel: w3035 -> [w3047 w3049 w3054]
                        tunnel: [w3046 w3048 w3052] -> w3030
                        tunnel: w3033 -> [w3045 _ _]
                        frame "nvarchar", Default {
                          n1777 = String Subset(string=w3047, length (rest)=w3045) -> (substring=w3046:string)  [unwired: 1 in]
                        }
                        frame "bit" {
                          n1778 = case shown="\"1\", \"T\", \"TRUE\"" w3049 {
                            tunnel: ["F" "T"] -> w3048
                            frame "False", Default {
                            }
                            frame "1", "T", "TRUE" {
                            }
                          }
                        }
                        frame "int" {
                          n1779 = Decimal String To Number(string=w3054) -> (number=w3053:i32)  [unwired: 2 in, 1 out]
                          n1780 = Number To Decimal String(number=w3053) -> (decimal integer string=w3052:string)  [unwired: 1 in]
                        }
                      }
                      n1781 = case shown="\"ComboBox\", \"String\", Default" w3032 {
                        tunnel: w3031 -> [_ w3041 w3044]
                        tunnel: w3030 -> [_ w3040 w3043]
                        frame "Boolean" {
                          # "Can Ignore"
                        }
                        frame "ComboBox", "String", Default {
                          n1782 = property class="Ctl"(reference=w3041, "Value"=w3040) -> ()  [unwired: 1 in, 2 out]
                        }
                        frame "Digital" {
                          n1783 = Decimal String To Number(string=w3043) -> (number=w3042:i32)  [unwired: 2 in, 1 out]
                          n1784 = property class="Ctl"(reference=w3044, "Value"=w3042) -> ()  [unwired: 1 in, 2 out]
                        }
                      }
                    }
                    frame -1 {
                    }
                  }
                }
                frame False {
                  # "Not Found. No Resize."
                }
              }
              n1785 = local read "Logon Extra"() -> (w2986:T25)
              n1786 = Unbundle By Name(w2986) -> ("IsUnicode"=w2985:bool)
              n1787 = case shown="True" w2985 {
                tunnel: w2990 -> [_ w3009]
                tunnel: w2989 -> [_ w3008]
                tunnel: w2988 -> [w3005 w3007]
                tunnel: [w3005 w3006] -> w2987
                frame False {
                }
                frame True {
                  # "isUnicode"
                  n1788 = case shown="\"String\"" w3009 {
                    tunnel: w3008 -> [w3014 _]
                    tunnel: w3007 -> [w3012 w3020]
                    tunnel: [w3011 w3020] -> w3006
                    frame "String" {
                      w3015 = refnum<vi> refnum  # String
                      # "Text.InterpAsUnicode\nSet after Logon"
                      # "Unicode - Set BOM to MCListbox"
                      n1789 = To More Specific Class(target class=w3015, reference=w3014) -> (specific class reference=w3013:refnum<vi>)  [unwired: 1 in, 1 out]
                      n1790 = property class="Str"(reference=w3013) -> ("Text.InterpretAsUnicode"=w3010:bool)  [unwired: 1 in, 2 out]
                      n1791 = case shown="True" w3010 {
                        tunnel: [w3016 w3018] -> w3011
                        tunnel: w3012 -> [w3016 w3017]
                        frame False {
                        }
                        frame True {
                          n1792 = Concatenate Strings("ÿþ", w3017) -> (w3018:string)
                        }
                      }
                    }
                    frame "Boolean", Default {
                    }
                  }
                }
              }
              n1793 = Replace Array Subset(array=w3003, new element=w2987, index (row)=w3001, index (col)=w3002) -> (w3000:string[][])
            }
            frame -1 {
            }
          }
        }
        n1794 = Decrement(x=w2831) -> (x-1=w2832:i32)
        n1795 = flat-sequence {
          tunnel: [w2892] -> w2828
          frame #0 {
            # "Uncheck empty Channel Mappings"
            n1796 = property on="Channel Mapping" class="Clust (strict)"() -> ("Value"=w2893:T2)  [unwired: 2 in, 2 out]
            n1797 = Cluster To Array(cluster=w2893) -> (array=w2894:string[])
            n1798 = for {
              tunnel: w2894 -> [w2899] mode=indexing
              tunnel: [w2896] -> w2889 mode=indexing
              n1799 = call <vilib>:"Trim Whitespace.vi"("string"=w2899) -> ("trimmed string"=w2898:string)  [unwired: 1 in]
              n1800 = Empty String/Path?(string/path=w2898) -> (empty?=w2897:bool)
              n1801 = Not(x=w2897) -> (.not. x?=w2896:bool)
            }
            n1802 = property on="Plot" class="Clust (strict)"() -> ("Value"=w2891:T4)  [unwired: 2 in, 2 out]
            n1803 = Cluster To Array(cluster=w2891) -> (array=w2890:bool[])
            n1804 = And(x=w2890, y=w2889) -> (x .and. y?=w2888:bool[])
            n1805 = Array To Cluster(array=w2888) -> (cluster=w2895:T69)
            n1806 = property on="Plot" class="Clust (strict)"("Value"=w2895) -> (error out=w2892:errorcluster)  [unwired: 2 in, 1 out]
          }
        }
        n1807 = case shown="1, Default" w2831 {
          tunnel: w2844 -> [_ w2907]
          tunnel: w2823 -> [_ w2906]
          tunnel: w2838 -> [_ w2905]
          tunnel: w2832 -> [_ w2904]
          tunnel: [FALSE w2903] -> w2830
          tunnel: ["" w2902] -> w2820
          frame 0 {
            # "No Mandatory Field"
          }
          frame 1, Default {
            # "At Least 1 Mandatory Field"
            n1808 = while {
              tunnel: w2907 -> [w2916]
              tunnel: w2905 -> [w2908] mode=indexing
              tunnel: w2906 -> [w2917]
              tunnel: [w2915] -> _
              tunnel: [w2914] -> _
              tunnel: w2904 -> [w2913]
              tunnel: [w2909] -> w2903
              tunnel: [w2908] -> w2902
              i -> [w2912]
              stop <- w2911 stop-if-true
              # "Check [IsMandatory] Fields"
              n1809 = Search 1D Array(1D array=w2916, element=w2908) -> (index of element=w2918:i32)  [unwired: 1 in]
              n1810 = Equal?(x=w2913, y=w2912) -> (x = y?=w2910:bool)
              n1811 = case shown="0, Default" w2918 {
                selector: w2918 -> [w2919 _]
                tunnel: w2917 -> [w2924 _]
                tunnel: [w2921 FALSE] -> w2909
                tunnel: [w2920 -1 ("index of element")] -> w2915
                tunnel: [w2919 -1 ("index of element")] -> w2914
                frame 0, Default {
                  # "Mandatory Field"
                  n1812 = Index Array(array=w2924, index (col)=w2919) -> (element=w2923:string[])  [unwired: 1 in]
                  n1813 = Search 1D Array(1D array=w2923, element="") -> (index of element=w2920:i32)  [unwired: 1 in]
                  n1814 = Greater Or Equal To 0?(x=w2920) -> (x >= 0?=w2921:bool)
                }
                frame -1 {
                }
              }
              n1815 = Or(x=w2909, y=w2910) -> (x .or. y?=w2911:bool)
            }
          }
        }
        "Empty String in Mandatory Field" <- w2830
        n1816 = control-ref of="Item Details"() -> (w2822:refnum<vi>)
        n1817 = property class="Clust (strict)"(reference=w2822) -> (error out=w2818:errorcluster, "Controls[]"=w2821:refnum<vi>[])  [unwired: 1 in, 1 out]
        n1818 = for {
          tunnel: w2821 -> [w2874] mode=indexing
          tunnel: w2820 -> [w2872]
          tunnel: [w2865] -> w2819
          tunnel: w2818 -> [w2870]
          tunnel: [w2869] -> w2817
          stop <- w2871 stop-if-true
          # "Get Caption of Part Details"
          n1819 = property class="Ctl"(reference=w2874, error in=w2870) -> (reference out=w2867:refnum<vi>, error out=w2869:errorcluster, "Label.Text"=w2873:string, "Caption.Text"=w2866:string, "ClassName"=w2868:string)
          n1820 = case shown="\"ComboBox\"" w2868 {
            tunnel: w2867 -> [_ w2881 w2887]
            tunnel: w2866 -> [w2875 w2877 w2883]
            tunnel: [w2875 w2876 w2882] -> w2865
            frame "False", Default {
            }
            frame "String" {
              w2880 = refnum<vi> refnum  # String
              n1821 = To More Specific Class(target class=w2880, reference=w2881) -> (specific class reference=w2879:refnum<vi>)  [unwired: 1 in, 1 out]
              n1822 = property class="Str"(reference=w2879) -> ("Text.InterpretAsUnicode"=w2878:bool)  [unwired: 1 in, 2 out]
              n1823 = call "String - Add BOM if IsUnicode.vi"("Input is Unicode (varbinary)?"=w2878, "String IN"=w2877) -> ("BOM Added"=w2876:string)  [unwired: 9 in]
            }
            frame "ComboBox" {
              w2886 = refnum<vi> refnum  # ComboBox
              n1824 = To More Specific Class(target class=w2886, reference=w2887) -> (specific class reference=w2885:refnum<vi>)  [unwired: 1 in, 1 out]
              n1825 = property class="CmbBox"(reference=w2885) -> ("Text.InterpretAsUnicode"=w2884:bool)  [unwired: 1 in, 2 out]
              n1826 = call "String - Add BOM if IsUnicode.vi"("Input is Unicode (varbinary)?"=w2884, "String IN"=w2883) -> ("BOM Added"=w2882:string)  [unwired: 9 in]
            }
          }
          n1827 = Equal?(x=w2873, y=w2872) -> (x = y?=w2871:bool)
        }
        n1828 = local write "Property Node Error"(w2817) -> ()
        n1829 = local read "Channel to Probe Mapping"() -> (w2841:cluster{"Channel to Probe Mapping":string})
        n1830 = Not(x=w2830) -> (.not. x?=w2829:bool)
        n1831 = Unbundle By Name(w2841) -> ("Channel to Probe Mapping"=w2840:string)
        n1832 = call "String - Channel to Probe Mappings.vi"("Channel to Probe Mapping"=w2840, "Channel to Probe Cluster Label"=w2843, "ColHdrString"=w2844, "ItemNames"=w2823) -> ("Probe List Valid"=w2826:bool, "Probe List"=→"Probe List":i32[], "Available Probe List"=w2827:string, "cRIO Channel List"=→"cRIO Channel List":i32[], "Duplicate"=w2825:bool, "Duplicated Probe #"=w2824:i32)  [unwired: 1 in, 1 out]
        "Probe List Valid" <- w2826
        n1833 = And(x=w2829, y=w2826) -> ()  [unwired: 1 out]
        n1834 = case shown="False" w2830 {
          tunnel: w2819 -> [_ w2960]
          tunnel: w2827 -> [w2936 _]
          tunnel: w2826 -> [w2935 _]
          tunnel: w2825 -> [w2934 _]
          tunnel: w2824 -> [w2933 _]
          tunnel: w2823 -> [w2932 _]
          frame False {
            # "No Empty Field"
            n1835 = case shown="False" w2935 {
              tunnel: w2936 -> [_ w2946]
              tunnel: w2934 -> [_ w2948]
              tunnel: w2933 -> [_ w2947]
              tunnel: w2932 -> [w2942 _]
              frame True {
                # "Insert to MCListBox"
                n1836 = property on="Order No." class="Str"() -> ("Value"=w2939:string)  [unwired: 2 in, 2 out]
                n1837 = property on="Part Details" class="MCListbox (strict)"("ItemNames"=w2942) -> ()  [unwired: 2 in, 2 out]
                n1838 = call "Msgbox - Message Handler.vi"("Short Description (When DB Not Available)"="Part Details Added" ("string"), "Description (When DB Not Available)"=" details added." ("string"), "Pre-Description"=w2939, "<.?....> Message Code"="<I 207>") -> ("MHandler Error"=w2941:errorcluster)  [unwired: 5 in, 2 out]
                n1839 = local write "MHandler"(w2941) -> ()
              }
              frame False {
                # "Probe List NOT valid. (Invalid Probe Number)"
                n1840 = case shown="True" w2948 {
                  tunnel: w2947 -> [_ w2958]
                  frame False {
                  }
                  frame True {
                    n1841 = Format Into String(format string="%d is duplicated. ", initial string="Probe Number ", w2958) -> ()  [unwired: 1 in, 2 out]
                  }
                }
                n1842 = Empty String/Path?(string/path=w2946) -> (empty?=w2945:bool)
                n1843 = case shown="False" w2945 {
                  tunnel: ["Please select from the following available probe no. :" ("string") "Please confirm current station is linked to the furnace."] -> w2949
                  tunnel: w2946 -> [_ _]
                  tunnel: ["<E 205>" ("<.?....> Message Code") "<E 204>" ("<.?....> Message Code")] -> w2944
                  tunnel: ["Invalid Probe Number. " ("string") "Probe Details Not Available. "] -> w2943
                  frame False {
                  }
                  frame True {
                    # "Empty Available Probe List"
                  }
                }
